vi "Write Configuration Parameter.vi"(8 "error in (no error)":errorcluster, 10 "Configuration":T1, 11 "ADAS PE Template in":refnum<class "ADAS PE Template.lvclass">) -> (0 "error out":errorcluster, 3 "ADAS PE Template out":refnum<class "ADAS PE Template.lvclass">)   [LabVIEW 2020, in "ADAS PE Template.lvlib" / "ADAS PE Template.lvclass"]
uses:
  ADAS PE Template.lvclass
  C:/Program Files/National Instruments/LabVIEW 2020/vi.lib/FlexLogger/SDK/PluginSDK.lvlibp/PEFClasses/SDK/Processing Element/Processing Element.lvclass
  Configuration.ctl
  Get Configuration Version.vi
  <vilib>/ADAS Record/Utilities/Config/Data Converter/Data Container and Version to JSON.vi
  <vilib>/FlexLogger/SDK/PluginSDK.lvlibp/PEFClasses/SDK/Processing Element/Read Parameters Property.vi
  <vilib>/FlexLogger/SDK/PluginSDK.lvlibp/PEFClasses/SDK/Parameters/Set Parameter.vi
  <vilib>/FlexLogger/SDK/PluginSDK.lvlibp/PEFClasses/SDK/Parameters/SetParameter(String).vi
  <vilib>/FlexLogger/SDK/PluginSDK.lvlibp/PEFClasses/SDK/Processing Element/Write Parameters Property.vi
  <vilib>/FlexLogger/SDK/PluginSDK.lvlibp/PEFClasses/SDK/Parameters/Parameters.lvclass
panel:
  # "#via_ignore"
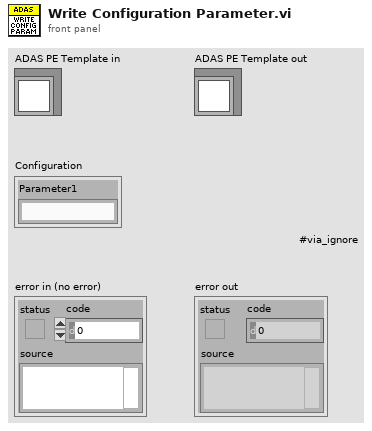
[diagram p1: front panel]
types:
  T1 = typedef "ADAS PE Template.lvlib/ADAS PE Template.lvclass/Configuration.ctl" = cluster{"Parameter1":string}
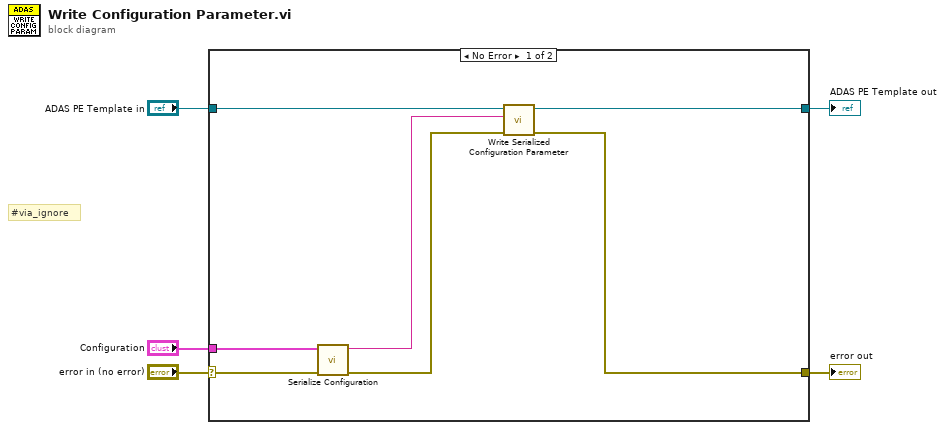
[diagram p0: block diagram]
diagram:
  # "#via_ignore"
  n1 = case shown="No Error" "error in (no error)" {
    selector: "error in (no error)" -> [w10 w14]
    tunnel: [w7 w14] -> w4
    tunnel: [w11 w13] -> w2
    tunnel: "ADAS PE Template in" -> [w12 w13]
    tunnel: "Configuration" -> [w6 _]
    frame No Error {
      n2 = call "Serialize Configuration.vi"("error in (no error)"=w10, "Configuration"=w6) -> ("error out"=w8:errorcluster, "Serialized Configuration"=w9:string)  [unwired: 8 in]
      n3 = call "Write Serialized Configuration Parameter.vi"("error in (no error)"=w8, "Serialized Configuration"=w9, "ADAS PE Template in"=w12) -> ("error out"=w7:errorcluster, "ADAS PE Template out"=w11:refnum<class "ADAS PE Template.lvclass">)  [unwired: 7 in]
    }
    frame Error {
    }
  }
  "error out" <- w4
  "ADAS PE Template out" <- w2
